vi "读取日数据.vi"(9 "table输入":string(combo), 10 "结束时间":string, 11 "起始时间":string) -> (0 "error out":errorcluster, 3 "data":string[][](table))   [LabVIEW 2016]
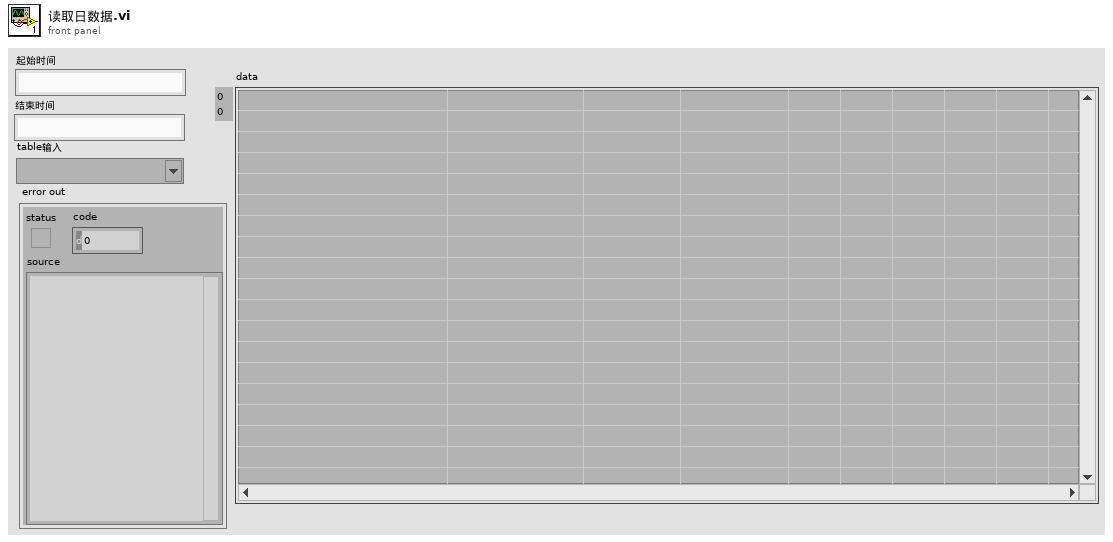
[diagram p1: front panel]
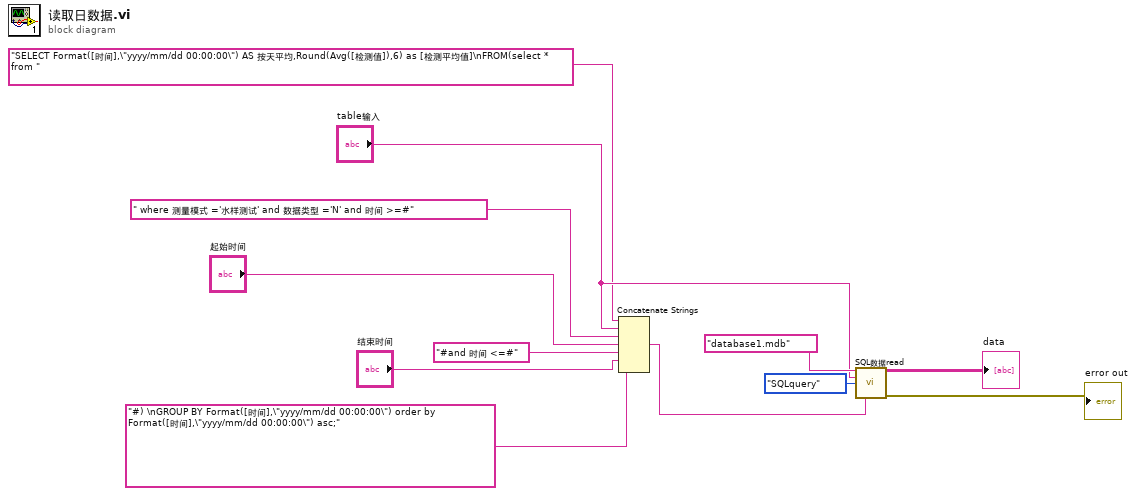
[diagram p0: block diagram]
diagram:
  n1 = Concatenate Strings("SELECT Format([时间],\"yyyy/mm/dd 00:00:00\") AS 按天平均,Round(Avg([检测值]),6) as [检测平均值]\nFROM(select * from ", "table输入", " where 测量模式 ='水样测试' and 数据类型 ='N' and 时间 >=#", "起始时间", "#and 时间 <=#", "结束时间", "#) \nGROUP BY Format([时间],\"yyyy/mm/dd 00:00:00\") order by Format([时间],\"yyyy/mm/dd 00:00:00\") asc;" ("字符串")) -> (w1:string)
  n2 = call "SQL数据read.vi"("database"="database1.mdb", "table输入"="table输入", "枚举"=enum16{"DBTOOL", "SQLquery"}."SQLquery", "SQL query"=w1) -> ("data"=→"data":string[][], "error out"=→"error out":errorcluster)  [unwired: 9 in, 1 out]
